vi "add2.vi"(8 "error in (no error)":errorcluster, 10 "startstop":bool, 11 "Status Actor in":refnum<class "Status Actor.lvclass">) -> (0 "error out":errorcluster, 3 "Status Actor out":refnum<class "Status Actor.lvclass">)   [LabVIEW 2019, in "Status Actor.lvlib" / "Status Actor.lvclass"]
uses:
  Status Actor.lvclass
  Status Actor.lvclass/Status Actor.ctl
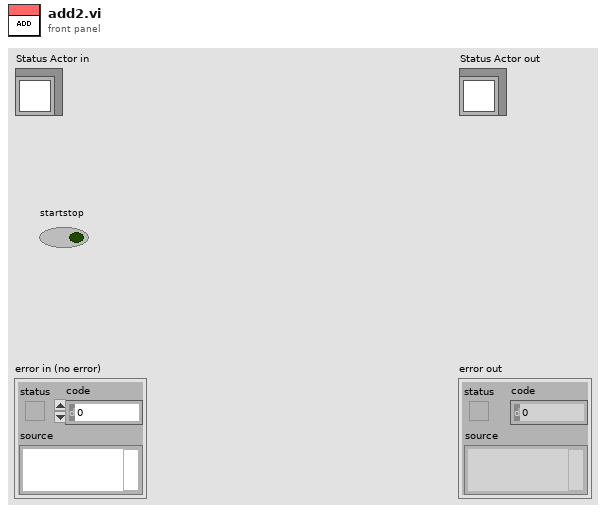
[diagram p1: front panel]
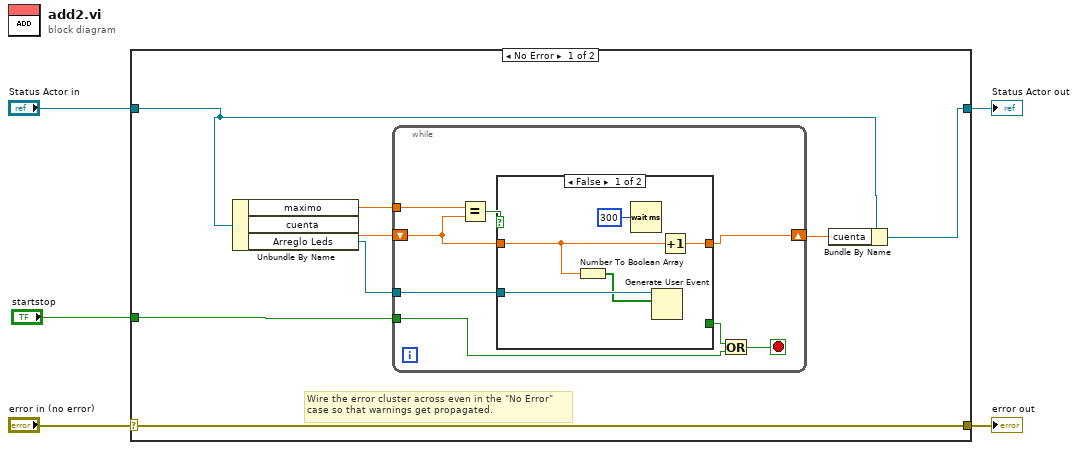
[diagram p0: block diagram]
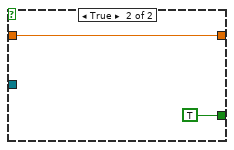
[diagram p2: hidden frame]
diagram:
  n1 = case shown="No Error" "error in (no error)" {
    selector: "error in (no error)" -> [w13 w30]
    tunnel: [w13 w30] -> w4
    tunnel: [w8 w29] -> w2
    tunnel: "Status Actor in" -> [w7 w29]
    tunnel: "startstop" -> [w6 _]
    frame No Error {
      # "Wire the error cluster across even in the \"No Error\"\ncase so that warnings get propagated."
      n2 = Unbundle By Name(w7) -> ("maximo"=w10:dbl, "cuenta"=w12:dbl, "Arreglo Leds"=w9:refnum<user-event>)
      n3 = while {
        tunnel: w10 -> [w18]
        tunnel: w9 -> [w17]
        shift-right: [w19] -> w11
        shift-left: w12 -> [w20]
        tunnel: w6 -> [w14]
        stop <- w15 stop-if-true
        n4 = Equal?(x=w18, y=w20) -> (x = y?=w21:bool)
        n5 = case shown="False" w21 {
          tunnel: w20 -> [w24 w28]
          tunnel: [w26 w28] -> w19
          tunnel: w17 -> [w25 _]
          tunnel: [_ TRUE] -> w16
          frame False {
            n6 = Number To Boolean Array(number=w24) -> (Boolean array=w23:bool[])
            n7 = Wait (ms)(milliseconds to wait=u32 300) -> ()  [unwired: 1 out]
            n8 = Generate User Event(user event=w25, event data cluster=w23) -> ()  [unwired: 2 in, 2 out]
            n9 = Increment(x=w24) -> (x+1=w26:dbl)
          }
          frame True {
          }
        }
        n10 = Or(x=w16, y=w14) -> (x .or. y?=w15:bool)
      }
      n11 = Bundle By Name(cluster=w7, "cuenta"=w11) -> (w8:refnum<class "Status Actor.lvclass">)
    }
    frame Error {
    }
  }
  "error out" <- w4
  "Status Actor out" <- w2
